vi "PH_Cont-601k_PSU.Action Set Voltage.vi"(0 "VI in":refnum<vi>, 2 "Voltage [V]":u16, 5 "error in (no error)":errorcluster) -> (14 "VI out":refnum<vi>, 19 "error out":errorcluster)   [LabVIEW 2014, in "PH_Cont-601k_PSU.lvlib"]
uses:
  PH_Cont-601k_PSU.lvlib
  PH_Cont-601k_PSU.Readyness Device.ctl
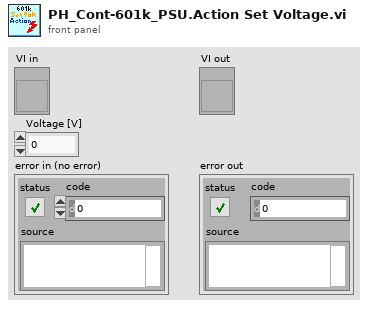
[diagram p1: front panel]
types:
  T1 = typedef "PH_Cont-601k_PSU.lvlib/PH_Cont-601k_PSU.Readyness Device.ctl" = enum32{"OFF", "CONNECTING", "CONNECTED", "OPERATING", "EOC", "ERROR"}
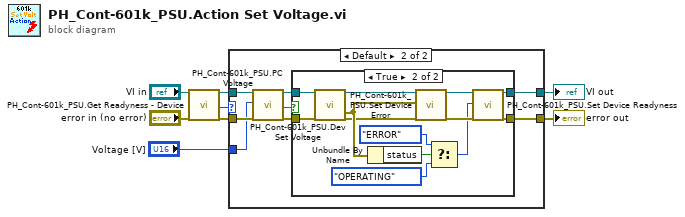
[diagram p0: block diagram]
diagram:
  n1 = call "PH_Cont-601k_PSU.Get Readyness - Device.vi"("VI in"="VI in", "error in (no error)"="error in (no error)") -> ("VI out"=w5:refnum<vi>, "Readyness - Device"=w8:T1, "error out"=w7:errorcluster)  [unwired: 15 in]
  n2 = case shown="Default" w8 {
    tunnel: [w9 w18] -> w2
    tunnel: [w10 w17] -> w3
    tunnel: w5 -> [w10 w16]
    tunnel: w7 -> [w9 w15]
    tunnel: "Voltage [V]" -> [_ w11]
    frame "OFF" {
    }
    frame Default {
      n3 = call "PH_Cont-601k_PSU.PC Voltage.vi"("VI in"=w16, "Voltage [V]"=w11, "error in (no error)"=w15) -> ("VI out"=w13:refnum<vi>, "\"Voltage\" changed"=w12:bool, "error out"=w14:errorcluster)  [unwired: 14 in]
      n4 = case shown="True" w12 {
        tunnel: w14 -> [w19 w33]
        tunnel: w13 -> [w20 w32]
        tunnel: [w20 w22] -> w17
        tunnel: [w19 w21] -> w18
        frame False {
        }
        frame True {
          n5 = call "PH_Cont-601k_PSU.Dev Set Voltage.vi"("VI in"=w32, "error in (no error)"=w33) -> ("VI out"=w24:refnum<vi>, "Device Error out"=w25:errorcluster, "error out"=w23:errorcluster)  [unwired: 15 in]
          n6 = Unbundle By Name(w25) -> ("status"=w27:bool)
          n7 = call "PH_Cont-601k_PSU.Set Device Error.vi"("VI in"=w24, "Device Error"=w25, "error in (no error)"=w23) -> ("VI out"=w30:refnum<vi>, "error out"=w31:errorcluster)  [unwired: 15 in]
          n8 = Select(t=PH_Cont-601k_PSU.Readyness_Device."ERROR" ("Readyness.Device"), s=w27, f=PH_Cont-601k_PSU.Readyness_Device."OPERATING" ("Readyness Device to set")) -> (s? t:f=w29:T1)
          n9 = call "PH_Cont-601k_PSU.Set Device Readyness.vi"("VI in"=w30, "Readyness Device to set"=w29, "error in (no error)"=w31) -> ("VI out"=w22:refnum<vi>, "error out"=w21:errorcluster)  [unwired: 15 in]
        }
      }
    }
  }
  "VI out" <- w3
  "error out" <- w2
